vi "FGV Timer.vi"(7 "Method (Get Time)":enum16{"Start", "Stop", "Reset", "Get Time"}(ring)=enum."Get Time", 8 "error in (no error)":errorcluster) -> (0 "error out":errorcluster, 2 "Running":bool, 3 "Elapsed Time (ms)":u32)   [LabVIEW 2011]
doc: "This is a functional global that acts as a timer in the same manner as a stopwatch. Use the Reset method to reset the timer. Start will start it. The user can stop and re - Start the timer. The Get Time method will return the elapsed time and the running status of the timer.\n\nAAL 9/09"
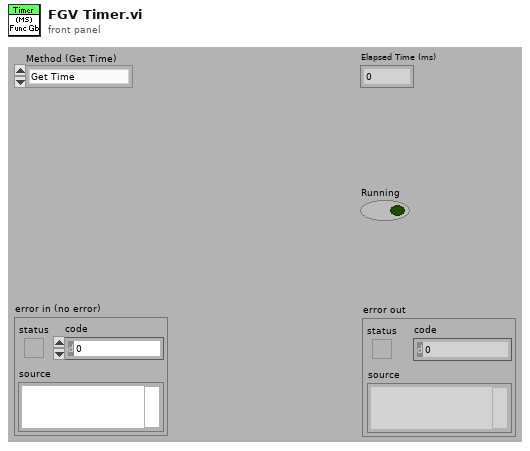
[diagram p1: front panel]
types:
  T1 = cluster{"Start Time":u32, "Elapsed Time":u32, "Running":bool}
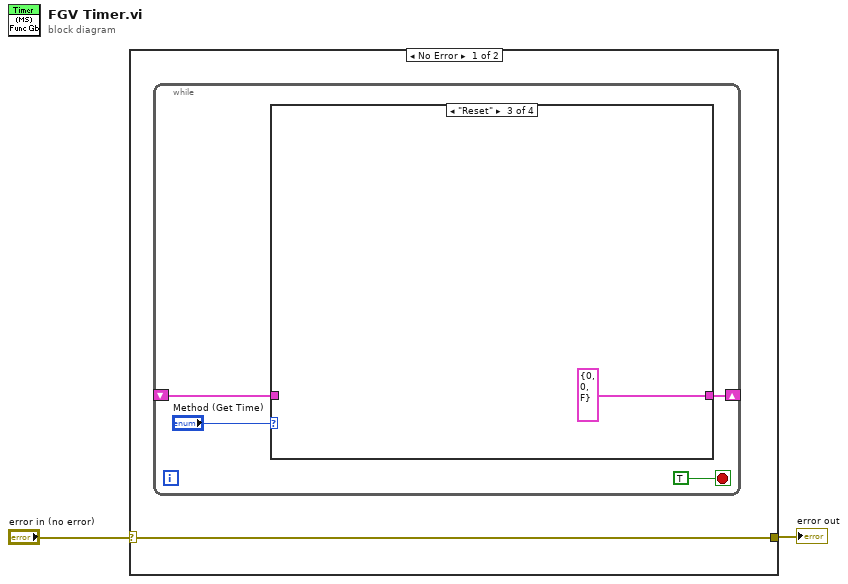
[diagram p0: block diagram]
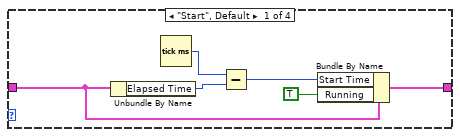
[diagram p2: hidden frame]
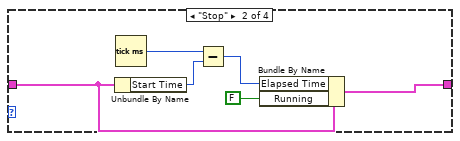
[diagram p3: hidden frame]
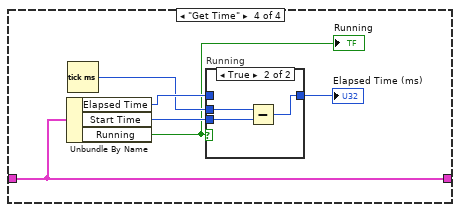
[diagram p4: hidden frame]
diagram:
  n1 = case shown="No Error" "error in (no error)" {
    selector: "error in (no error)" -> [w3 w31]
    tunnel: [w3 w31] -> w1
    frame No Error {
      n2 = while {
        shift-right: [w6] -> _
        shift-left: _ -> [w5]
        stop <- TRUE stop-if-true
        n3 = case shown="\"Reset\"" "Method (Get Time)" {
          tunnel: [w8 w14 T1 {"Start Time"=0, "Elapsed Time"=0, "Running"=FALSE} w23] -> w6
          tunnel: w5 -> [w9 w15 _ w23]
          frame "Start", Default {
            n4 = Unbundle By Name(w9) -> ("Elapsed Time"=w11:u32)
            n5 = Tick Count (ms)() -> (millisecond timer value=w10:u32)
            n6 = Subtract(x=w10, y=w11) -> (x-y=w12:u32)
            n7 = Bundle By Name(cluster=w9, "Start Time"=w12, "Running"=TRUE) -> (w8:T1)
          }
          frame "Stop" {
            n8 = Unbundle By Name(w15) -> ("Start Time"=w17:u32)
            n9 = Tick Count (ms)() -> (millisecond timer value=w16:u32)
            n10 = Subtract(x=w16, y=w17) -> (x-y=w19:u32)
            n11 = Bundle By Name(cluster=w15, "Elapsed Time"=w19, "Running"=FALSE) -> (w14:T1)
          }
          frame "Reset" {
          }
          frame "Get Time" {
            n12 = Unbundle By Name(w23) -> ("Elapsed Time"=w26:u32, "Start Time"=w25:u32, "Running"=w22:bool)
            "Running" <- w22
            n13 = Tick Count (ms)() -> (millisecond timer value=w24:u32)
            n14 = case "Running" shown="True" w22 {
              tunnel: w24 -> [_ w30]
              tunnel: w25 -> [_ w29]
              tunnel: [w27 w28] -> w21
              tunnel: w26 -> [w27 _]
              frame False {
              }
              frame True {
                n15 = Subtract(x=w30, y=w29) -> (x-y=w28:u32)
              }
            }
            "Elapsed Time (ms)" <- w21
          }
        }
      }
    }
    frame Error {
    }
  }
  "error out" <- w1
